vi "Exit Initialize (User).vi"(8 "error in":errorcluster, 11 "Node in":refnum<class "ThermotronDriver.lvclass">) -> (0 "error out":errorcluster, 3 "Node out":refnum<class "ThermotronDriver.lvclass">)   [LabVIEW 2023, in "ThermotronDriver.lvlib" / "ThermotronDriver.lvclass"]
uses:
  ThermotronDriver.lvclass
  ThermotronDriver.lvclass/ThermotronDriver.ctl
  Support/LabVIEW API/Thermotron8800InstrumentDriver64bitForLabView2018/Thermotron 8800/Thermotron 8800.lvlib
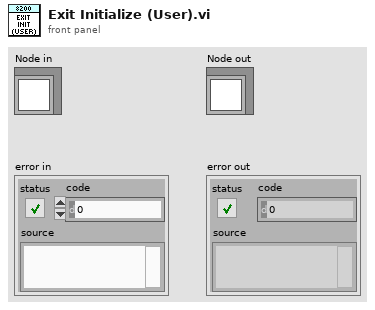
[diagram p1: front panel]
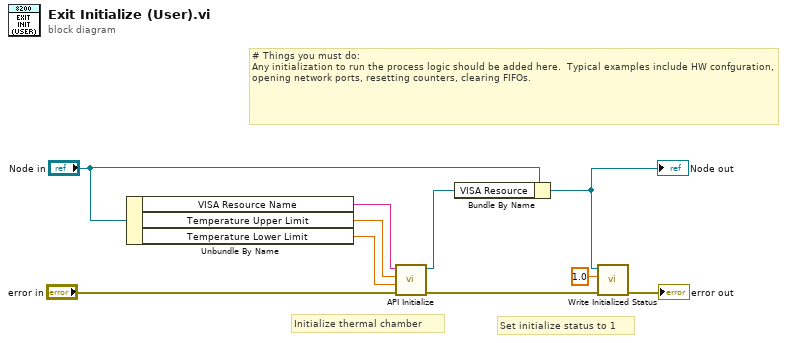
[diagram p0: block diagram]
diagram:
  # "Set initialize status to 1"
  # "Initialize thermal chamber"
  # "# Things you must do:\nAny initialization to run the process logic should be added here.  Typical examples include HW confguration, opening network ports, resetting counters, clearing FIFOs."
  n1 = Unbundle By Name("Node in") -> ("VISA Resource Name"=w9:string, "Temperature Upper Limit"=w8:dbl, "Temperature Lower Limit"=w7:dbl)
  n2 = call "API Initialize.vi"("error in (no error)"="error in", "Temperature Lower Limit"=w7, "Temperature Upper Limit"=w8, "VISA resource name"=w9) -> ("error out"=w6:errorcluster, "VISA resource out"=w2:refnum<visa-resource-name>)  [unwired: 6 in]
  n3 = Bundle By Name(cluster="Node in", "VISA Resource"=w2) -> (w1:refnum<class "ThermotronDriver.lvclass">)
  "Node out" <- w1
  n4 = call-dynamic "Write Initialized Status.vi"("error in (no error)"=w6, "Initialized Status"=1.0, "ThermotronDriver in"=w1) -> ("error out"=→"error out":errorcluster)  [unwired: 7 in, 1 out]
